vi "HEWH Draw End Clean Up.vi"(5 "Test Data-Start to End DBL":dbl[][](array[numeric]), 6 "Draw Start":i32, 7 "Totalized Flow Index":i32, 8 "error in (no error)":errorcluster, 9 "Sub Array End Index":i32, 10 "Rate":dbl[](array[numeric]), 11 "Total":dbl[](array[numeric])) -> (0 "error out":errorcluster, 2 "Numeric":i32, 3 "Test Data-Start to End DBL Output":dbl[][](array[numeric]))   [LabVIEW 2019]
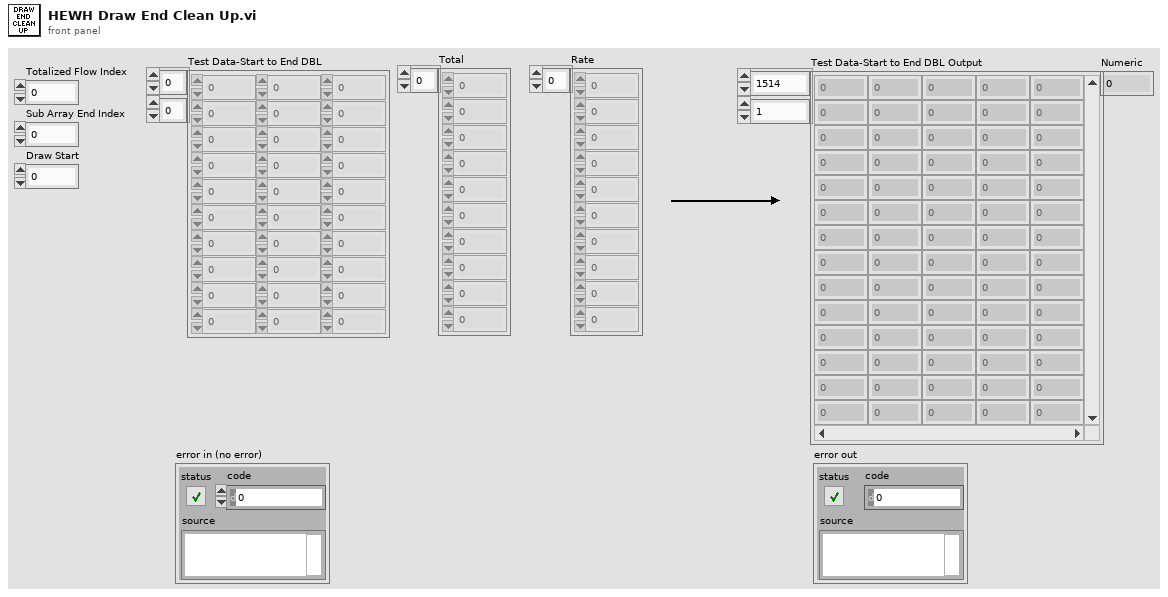
[diagram p1: front panel]
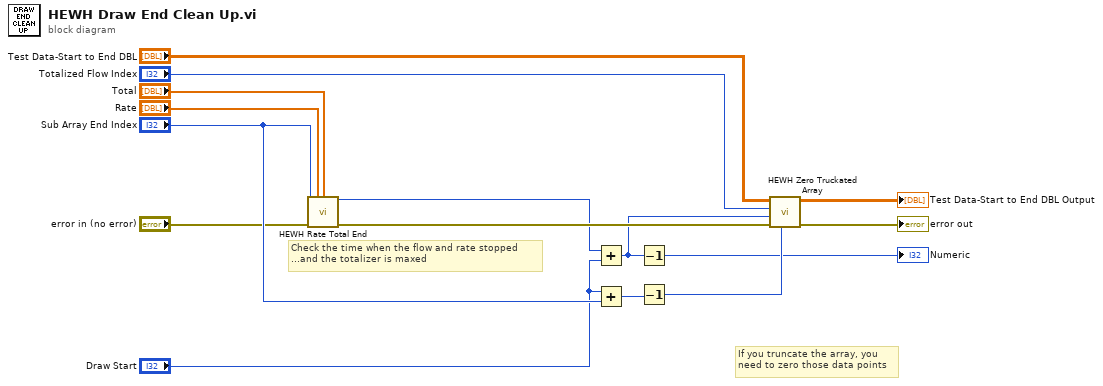
[diagram p0: block diagram]
diagram:
  # "If you truncate the array, you\nneed to zero those data points"
  # "Check the time when the flow and rate stopped\n...and the totalizer is maxed"
  n1 = call "HEWH Rate Total End.vi"("Sub Array End Index in"="Sub Array End Index", "Rate"="Rate", "Total"="Total", "error in (no error)"="error in (no error)") -> ("Sub Array Out"=w7:i32, "error out"=w13:errorcluster)  [unwired: 10 in]
  n2 = Add(x=w7, y="Draw Start") -> (x+y=w6:i32)
  n3 = Add(x="Draw Start", y="Sub Array End Index") -> (x+y=w9:i32)
  n4 = Decrement(x=w6) -> (x-1=→"Numeric":i32)
  n5 = Decrement(x=w9) -> (x-1=w12:i32)
  n6 = call "HEWH Zero Truckated Array.vi"("Zero End Index"=w12, "error in (no error)"=w13, "Zero Start Index"=w6, "Totalized Flow Index"="Totalized Flow Index", "Test Data-Start to End DBL"="Test Data-Start to End DBL") -> ("error out"=→"error out":errorcluster, "Test Data-Start to End DBL Output"=→"Test Data-Start to End DBL Output":dbl[][])  [unwired: 5 in]
